vi "retinotopic_map_display_only_120520.vi"() -> ()   [LabVIEW 2019]
uses:
  <vilib>/Utility/file.llb/Write Delimited Spreadsheet (DBL).vi
panel:
  out "Output":dbl[][](array[numeric])
  out "Display":bool=TRUE
  out "Trial":u32=1
  out "Stimuli Loaded?":bool
  out "Horizontal":bool
  out "stim_id":dbl[](array[numeric])
  out "Vertical":bool
  out "stim_loaded":dbl
  out "Elapsed Time":dbl
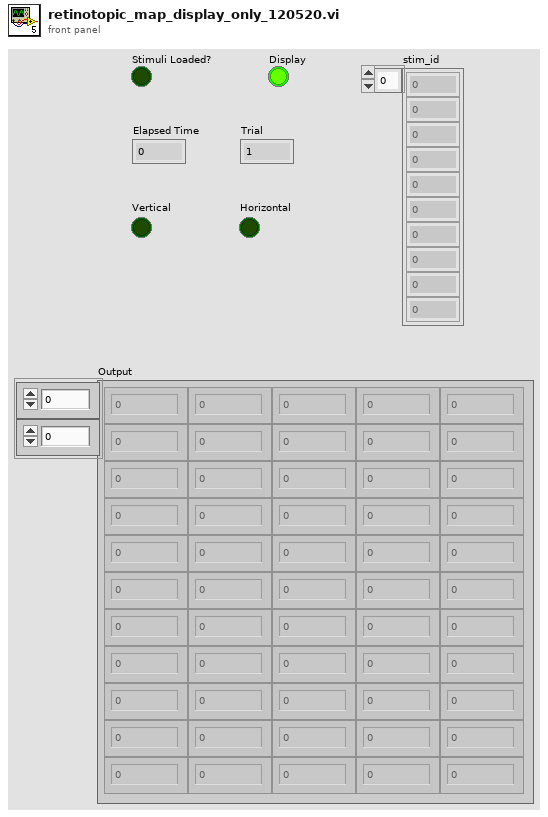
[diagram p1: front panel]
types:
  T1 = typedef "NI_Matrix.lvlib/RealMatrix.ctl" = dbl[][]
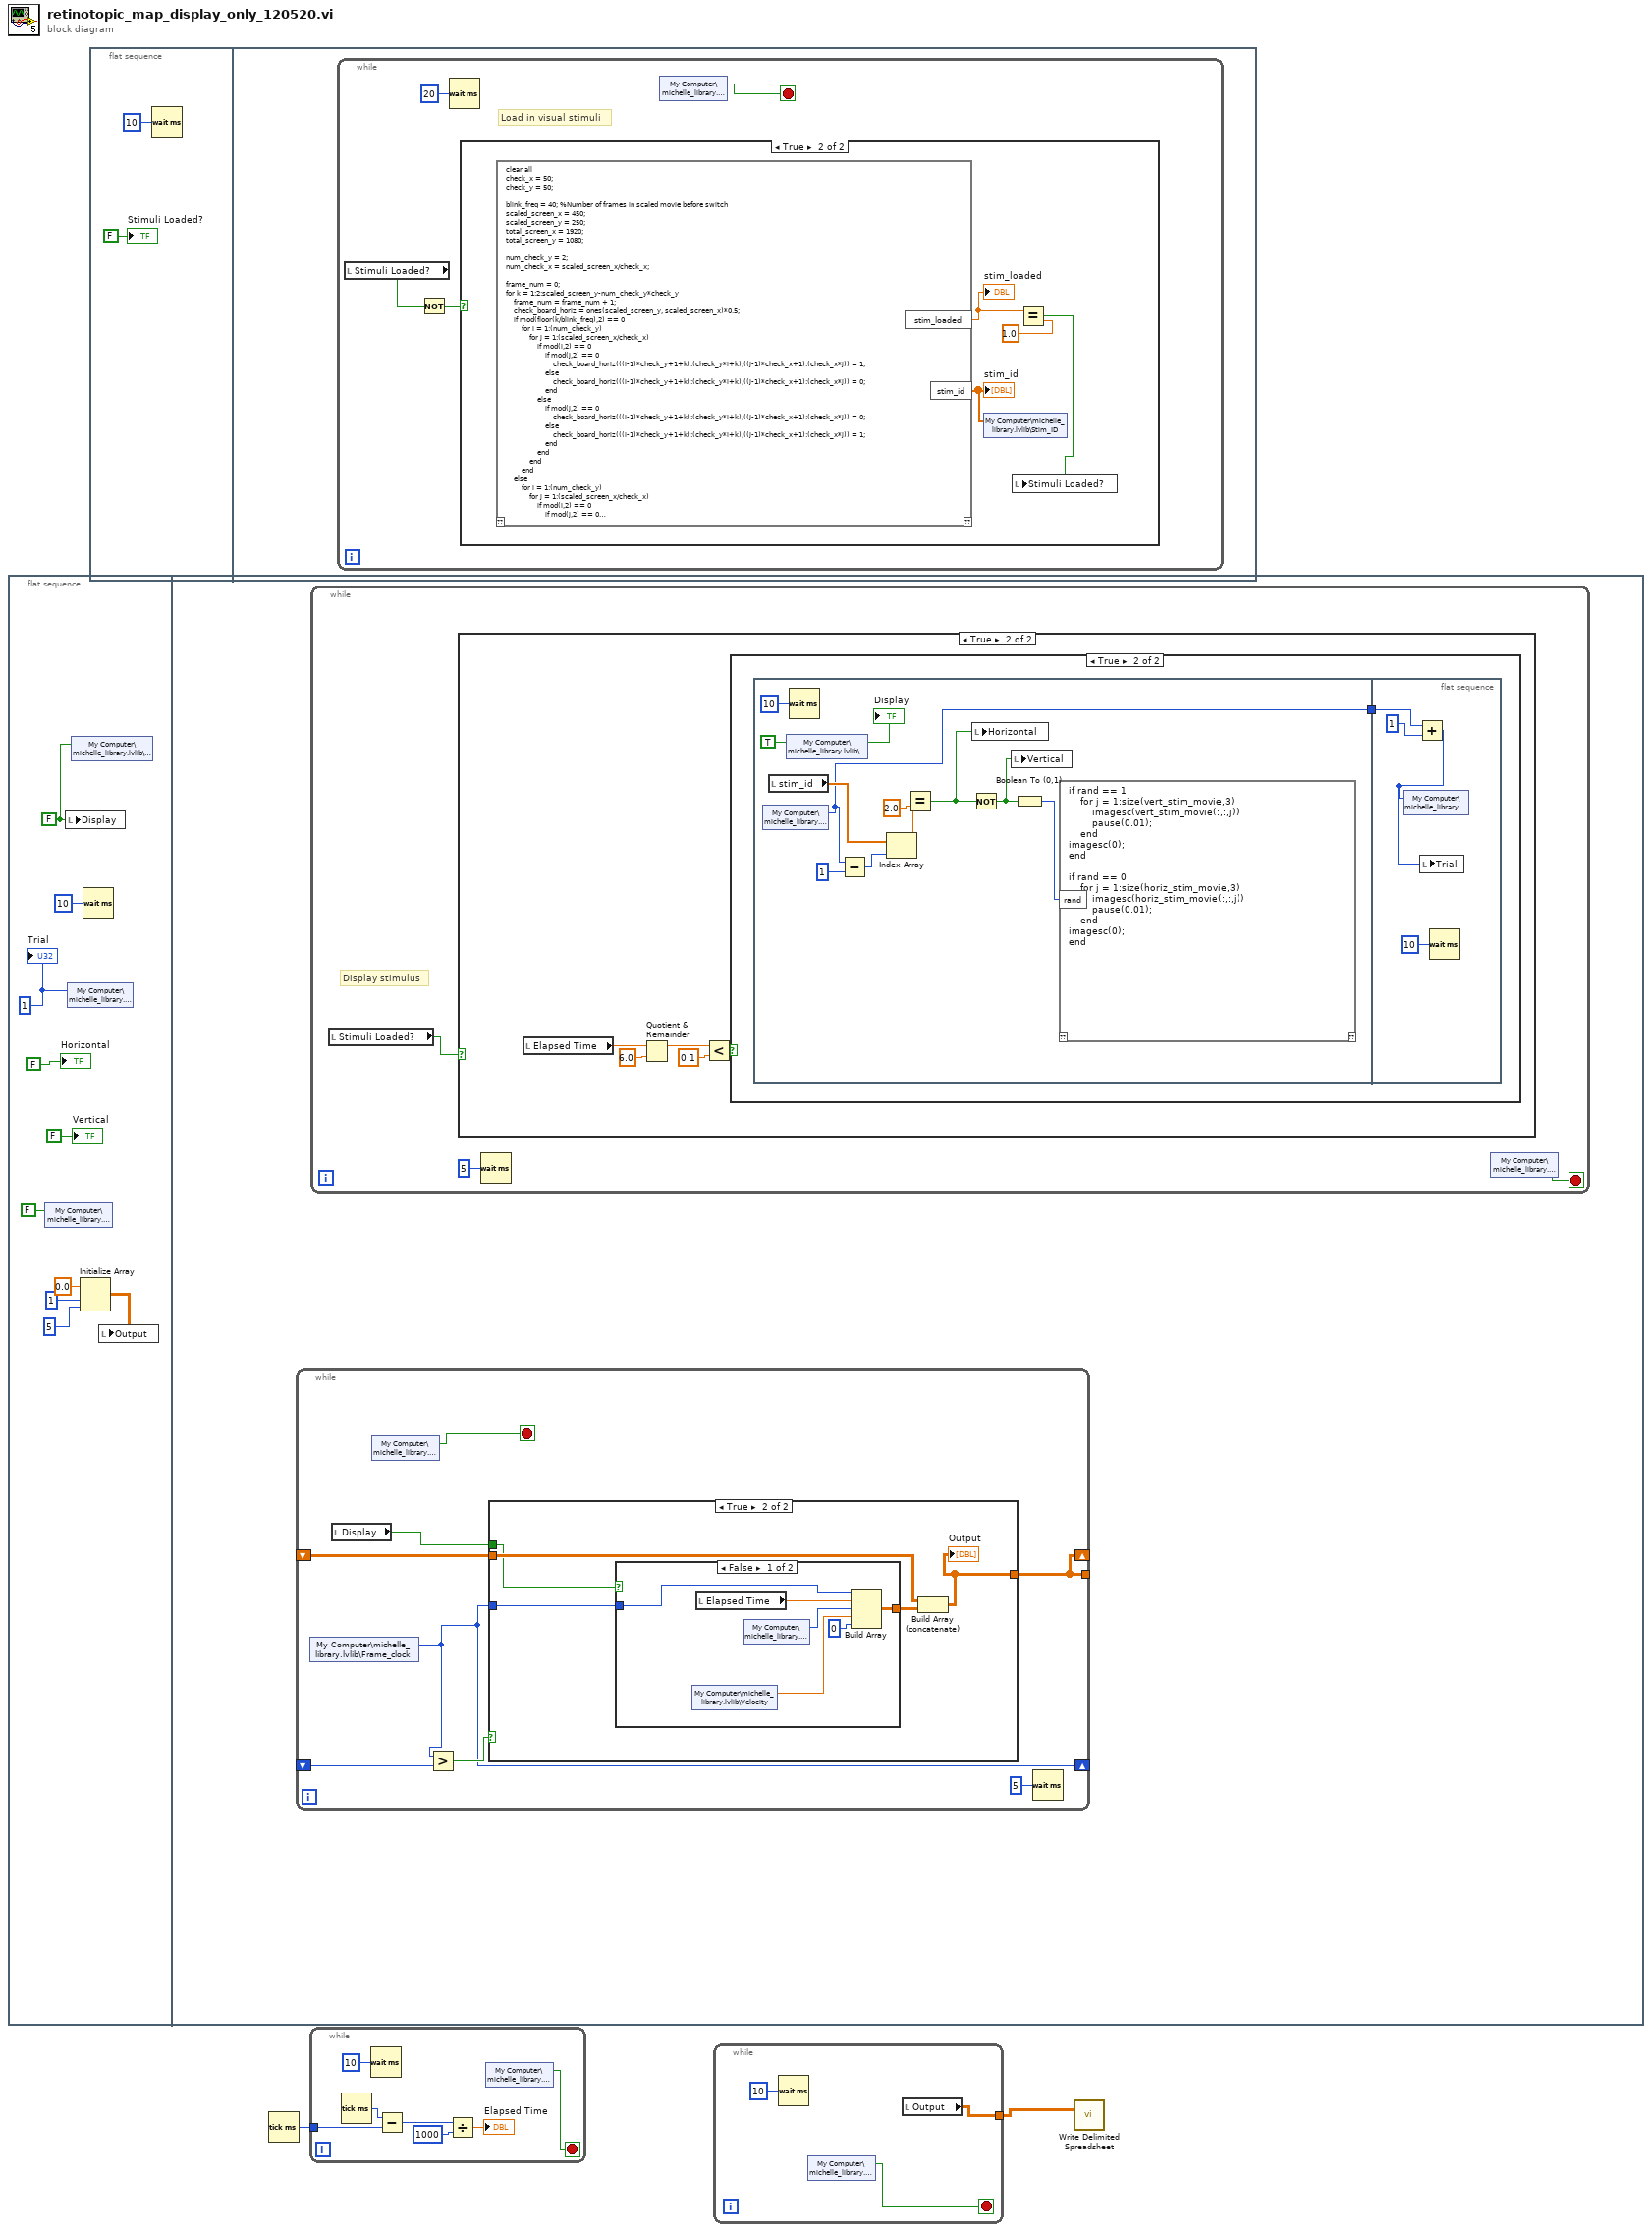
[diagram p0: block diagram]
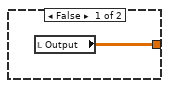
[diagram p3: hidden frame]
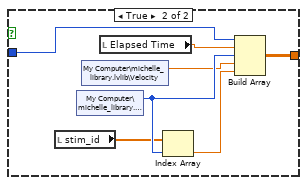
[diagram p4: hidden frame]
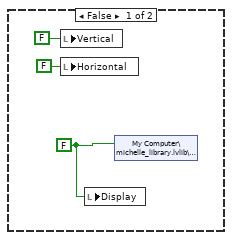
[diagram p6: hidden frame]
diagram:
  n1 = flat-sequence {
    frame #0 {
      w8 = FALSE ("Display")
      w12 = u32 1 ("Trial")
      n2 = shared-variable "My Computer\\michelle_library.lvlib\\Stop"(FALSE ("Stop")) -> ()  [unwired: 1 in, 1 out]
      n3 = local write "Display"(w8) -> ()
      n4 = shared-variable "My Computer\\michelle_library.lvlib\\Trial"(w12) -> ()  [unwired: 1 in, 1 out]
      n5 = shared-variable "My Computer\\michelle_library.lvlib\\Display"(w8) -> ()  [unwired: 1 in, 1 out]
      n6 = Initialize Array(0.0 ("element"), 1 ("dimension size"), 5 ("dimension size")) -> (w4:dbl[][])
      n7 = Wait (ms)(milliseconds to wait=u32 10) -> ()  [unwired: 1 out]
      n8 = local write "Output"(w4) -> ()
      "Horizontal" <- FALSE ("Stimulus 2")
      "Vertical" <- FALSE ("Stimulus 1")
      "Trial" <- w12
    }
    frame #1 {
      n9 = while {
        shift-right: [w15] -> _
        shift-left: _ -> [w20]
        shift-right: [w16] -> _
        shift-left: _ -> [w18]
        tunnel: [w16] -> _
        stop <- w14 stop-if-true
        n10 = shared-variable "My Computer\\michelle_library.lvlib\\Frame_clock"() -> (w15:u32)  [unwired: 1 in, 1 out]
        n11 = local read "Display"() -> (w13:bool)
        n12 = shared-variable "My Computer\\michelle_library.lvlib\\Stop"() -> (w14:bool)  [unwired: 1 in, 1 out]
        n13 = Greater?(x=w15, y=w20) -> (0:w19:bool)
        n14 = case shown="True" w19 {
          tunnel: w15 -> [_ w26]
          tunnel: w18 -> [_ w25]
          tunnel: [w21 w22] -> w16
          tunnel: w13 -> [_ w23]
          frame False {
            n15 = local read "Output"() -> (w21:dbl[][])
          }
          frame True {
            n16 = case shown="False" w23 {
              tunnel: w26 -> [w28 w39]
              tunnel: [w31 w38] -> w24
              frame False {
                n17 = shared-variable "My Computer\\michelle_library.lvlib\\Velocity"() -> (w27:dbl)  [unwired: 1 in, 1 out]
                n18 = local read "Elapsed Time"() -> (w30:dbl)
                n19 = shared-variable "My Computer\\michelle_library.lvlib\\Trial"() -> (w29:u32)  [unwired: 1 in, 1 out]
                n20 = Build Array(w28, w30, w29, w27, 0) -> (w31:T1)
              }
              frame True {
                n21 = local read "stim_id"() -> (w33:dbl[])
                n22 = shared-variable "My Computer\\michelle_library.lvlib\\Trial"() -> (w36:u32)  [unwired: 1 in, 1 out]
                n23 = shared-variable "My Computer\\michelle_library.lvlib\\Velocity"() -> (w34:dbl)  [unwired: 1 in, 1 out]
                n24 = local read "Elapsed Time"() -> (w37:dbl)
                n25 = Index Array(array=w33, index=w36) -> (element=w35:dbl)
                n26 = Build Array(w39, w37, w36, w34, w35) -> (w38:T1)
              }
            }
            n27 = Build Array (concatenate)(w25, w24) -> (w22:T1)
            "Output" <- w22
          }
        }
        n28 = Wait (ms)(milliseconds to wait=u32 5) -> ()  [unwired: 1 out]
      }
      n29 = while {
        stop <- w41 stop-if-true
        # "Display stimulus"
        n30 = local read "Stimuli Loaded?"() -> (w40:bool)
        n31 = case shown="True" w40 {
          frame False {
          }
          frame True {
            n32 = local read "Elapsed Time"() -> (w47:dbl)
            n33 = Quotient & Remainder(x=w47, y=6.0) -> (x-y*floor(x/y)=w45:dbl)  [unwired: 1 out]
            n34 = Less?(x=w45, y=0.1) -> (x < y?=w43:bool)
            n35 = case shown="True" w43 {
              frame False {
                w48 = FALSE ("Display")
                n36 = local write "Vertical"(FALSE) -> ()
                n37 = local write "Horizontal"(FALSE ("Horizontal")) -> ()
                n38 = local write "Display"(w48) -> ()
                n39 = shared-variable "My Computer\\michelle_library.lvlib\\Display"(w48) -> ()  [unwired: 1 in, 1 out]
              }
              frame True {
                n40 = flat-sequence {
                  tunnel: [w53] -> w51
                  tunnel: w51 -> [w66]
                  frame #0 {
                    w57 = TRUE ("Boolean")
                    n41 = shared-variable "My Computer\\michelle_library.lvlib\\Trial"() -> (w53:u32)  [unwired: 1 in, 1 out]
                    n42 = local read "stim_id"() -> (w61:dbl[])
                    n43 = shared-variable "My Computer\\michelle_library.lvlib\\Display"(w57) -> ()  [unwired: 1 in, 1 out]
                    n44 = Wait (ms)(milliseconds to wait=u32 10) -> ()  [unwired: 1 out]
                    n45 = Subtract(x=w53, y=u32 1) -> (x-y=w54:u32)
                    n46 = Index Array(array=w61, index=w54) -> (element=w60:dbl)
                    n47 = Equal?(x=w60, y=2.0) -> (x = y?=w58:bool)
                    n48 = Not(x=w58) -> (.not. x?=w55:bool)
                    n49 = local write "Horizontal"(w58) -> ()
                    n50 = local write "Vertical"(w55) -> ()
                    n51 = Boolean To (0,1)(Boolean=w55) -> (0, 1=w56:i16)
                    n52 = script code="if rand == 1\n    for j = 1:size(vert_stim_movie,3)\n        imagesc(vert_stim_movie(:,:,j))\n        pause(0.01);\n    end\nimagesc(0);\nend\n\nif rand == 0\n    for j = 1:size(horiz_stim_movie,3)\n        imagesc(horiz_stim_movie(:,:,j))\n        pause(0.01);\n    end\nimagesc(0);\nend"("rand"=w56) -> ()  [unwired: 1 in, 1 out]
                    "Display" <- w57
                  }
                  frame #1 {
                    n53 = Add(x=w66, y=u32 1) -> (x+y=w64:u32)
                    n54 = shared-variable "My Computer\\michelle_library.lvlib\\Trial"(w64) -> ()  [unwired: 1 in, 1 out]
                    n55 = local write "Trial"(w64) -> ()
                    n56 = Wait (ms)(milliseconds to wait=u32 10) -> ()  [unwired: 1 out]
                  }
                }
              }
            }
          }
        }
        n57 = Wait (ms)(milliseconds to wait=u32 5) -> ()  [unwired: 1 out]
        n58 = shared-variable "My Computer\\michelle_library.lvlib\\Stop"() -> (w41:bool)  [unwired: 1 in, 1 out]
      }
    }
  }
  n59 = flat-sequence {
    frame #0 {
      n60 = Wait (ms)(milliseconds to wait=u32 10) -> ()  [unwired: 1 out]
      "Stimuli Loaded?" <- FALSE ("Stimuli Loaded?")
    }
    frame #1 {
      n61 = while {
        stop <- w70 stop-if-true
        # "Load in visual stimuli"
        n62 = local read "Stimuli Loaded?"() -> (w69:bool)
        n63 = Not(x=w69) -> (.not. x?=w72:bool)
        n64 = Wait (ms)(milliseconds to wait=u32 20) -> ()  [unwired: 1 out]
        n65 = case shown="True" w72 {
          frame False {
          }
          frame True {
            n66 = script code="clear all\ncheck_x = 50;\ncheck_y = 50;\n\nblink_freq = 40; %Number of frames in scaled movie before switch\nscaled_screen_x = 450;\nscaled_screen_y = 250;\ntotal_screen_x = 1920;\ntotal_screen_y = 1080;\n\nnum_check_y = 2;\nnum_check_x = scaled_screen_x/check_x;\n\nframe_num = 0;\nfor k = 1:2:scaled_screen_y-num_check_y*check_y\n    frame_num = frame_num + 1;\n    check_board_horiz = ones(scaled_screen_y, scaled_screen_x)*0.5;\n    if mod(floor(k/blink_freq),2) == 0\n        for i = 1:(num_check_y)\n            for j = 1:(scaled_screen_x/check_x)\n                if mod(i,2) == 0\n                    if mod(j,2) == 0\n                        check_board_horiz(((i-1)*check_y+1+k):(check_y*i+k),((j-1)*check_x+1):(check_x*j)) = 1;\n                    else\n                        check_board_horiz(((i-1)*check_y+1+k):(check_y*i+k),((j-1)*check_x+1):(check_x*j)) = 0;\n                    end\n                else\n                    if mod(j,2) == 0\n                        check_board_horiz(((i-1)*check_y+1+k):(check_y*i+k),((j-1)*check_x+1):(check_x*j)) = 0;\n                    else\n                        check_board_horiz(((i-1)*check_y+1+k):(check_y*i+k),((j-1)*check_x+1):(check_x*j)) = 1;\n                    end\n                end\n            end\n        end\n    else\n        for i = 1:(num_check_y)\n            for j = 1:(scaled_screen_x/check_x)\n                if mod(i,2) == 0\n                    if mod(j,2) == 0\n                        check_board_horiz(((i-1)*check_y+1+k):(check_y*i+k),((j-1)*check_x+1):(check_x*j)) = 0;\n                    else\n                        check_board_horiz(((i-1)*check_y+1+k):(check_y*i+k),((j-1)*check_x+1):(check_x*j)) = 1;\n                    end\n                else\n                    if mod(j,2) == 0\n                        check_board_horiz(((i-1)*check_y+1+k):(check_y*i+k),((j-1)*check_x+1):(check_x*j)) = 1;\n                    else\n                        check_board_horiz(((i-1)*check_y+1+k):(check_y*i+k),((j-1)*check_x+1):(check_x*j)) = 0;\n                    end\n                end\n            end\n        end\n    end\n    horiz_stim_movie(:,:,frame_num) = check_board_horiz;\nend\n\nnum_check_y = scaled_screen_y/check_y;\nnum_check_x = 2;\n\nframe_num = 0;\nfor k = 1:2:scaled_screen_x-num_check_x*check_x\n    frame_num = frame_num + 1;\n    check_board_vert = ones(scaled_screen_y, scaled_screen_x)*0.5;\n    if mod(floor(k/blink_freq),2) == 0\n        for i = 1:(num_check_x)\n            for j = 1:(scaled_screen_y/check_y)\n                if mod(i,2) == 0\n                    if mod(j,2) == 0\n                        check_board_vert(((j-1)*check_y+1):check_y*j,((i-1)*check_x+1+k):(check_x*i+k)) = 1;\n                    else\n                        check_board_vert(((j-1)*check_y+1):check_y*j,((i-1)*check_x+1+k):(check_x*i+k)) = 0;\n                    end\n                else\n                    if mod(j,2) == 0\n                        check_board_vert(((j-1)*check_y+1):check_y*j,((i-1)*check_x+1+k):(check_x*i+k)) = 0;\n                    else\n                        check_board_vert(((j-1)*check_y+1):check_y*j,((i-1)*check_x+1+k):(check_x*i+k)) = 1;\n                    end\n                end\n            end\n        end\n    else\n        for i = 1:(num_check_x)\n            for j = 1:(scaled_screen_y/check_y)\n                if mod(i,2) == 0\n                    if mod(j,2) == 0\n                        check_board_vert(((j-1)*check_y+1):check_y*j,((i-1)*check_x+1+k):(check_x*i+k)) = 0;\n                    else\n                        check_board_vert(((j-1)*check_y+1):check_y*j,((i-1)*check_x+1+k):(check_x*i+k)) = 1;\n                    end\n                else\n                    if mod(j,2) == 0\n                        check_board_vert(((j-1)*check_y+1):check_y*j,((i-1)*check_x+1+k):(check_x*i+k)) = 1;\n                    else\n                        check_board_vert(((j-1)*check_y+1):check_y*j,((i-1)*check_x+1+k):(check_x*i+k)) = 0;\n                    end\n                end\n            end\n        end\n    end\n    vert_stim_movie(:,:,frame_num) = check_board_vert;\nend\n\nset(0, 'DefaultFigurePosition', [1914 0 1940 2000]);\ncolormap(gray(256))\nset(gcf,'MenuBar','none')\nset(gca,'DataAspectRatioMode','auto')\nset(gca,'Position',[0 0 1 1])\nset(gca, 'xlimmode','manual',...\n           'ylimmode','manual',...\n           'zlimmode','manual',...\n           'climmode','manual',...\n           'alimmode','manual');\nimshow(zeros(total_screen_y,total_screen_x))\n\nstim_id = [ones(1,210)];\naltern = [1:105]*2;\nstim_id(altern) = 2;\nstim_loaded = 1;"() -> ("stim_loaded"=w76:dbl, "stim_id"=w74:dbl[])  [unwired: 1 in, 1 out]
            "stim_loaded" <- w76
            "stim_id" <- w74
            n67 = shared-variable "My Computer\\michelle_library.lvlib\\Stim_ID"(w74) -> ()  [unwired: 1 in, 1 out]
            n68 = Equal?(x=w76, y=1.0) -> (x = y?=w73:bool)
            n69 = local write "Stimuli Loaded?"(w73) -> ()
          }
        }
        n70 = shared-variable "My Computer\\michelle_library.lvlib\\Stop"() -> (w70:bool)  [unwired: 1 in, 1 out]
      }
    }
  }
  n71 = Tick Count (ms)() -> (millisecond timer value=w2:u32)
  n72 = while {
    tunnel: w2 -> [w80]
    stop <- w77 stop-if-true
    n73 = Tick Count (ms)() -> (millisecond timer value=w81:u32)
    n74 = Wait (ms)(milliseconds to wait=u32 10) -> ()  [unwired: 1 out]
    n75 = Subtract(x=w81, y=w80) -> (x-y=w78:u32)
    n76 = Divide(x=w78, y=u32 1000) -> (x/y=→"Elapsed Time":dbl)
    n77 = shared-variable "My Computer\\michelle_library.lvlib\\Stop"() -> (w77:bool)  [unwired: 1 in, 1 out]
  }
  n78 = while {
    tunnel: [w84] -> w1
    stop <- w86 stop-if-true
    n79 = Wait (ms)(milliseconds to wait=u32 10) -> ()  [unwired: 1 out]
    n80 = shared-variable "My Computer\\michelle_library.lvlib\\Stop"() -> (w86:bool)  [unwired: 1 in, 1 out]
    n81 = local read "Output"() -> (w84:dbl[][])
  }
  n82 = call-poly <vilib>:"Write Delimited Spreadsheet.vi"("2D data"=w1) -> ()  [unwired: 13 in, 2 out]
